vi "Init.vi"(8 "error in":errorcluster) -> (0 "error out":errorcluster)   [LabVIEW 2018, in "UDP Writer.lvlib"]
doc: "This subVI enqueues the named action in to the communications queue along with the input data."
uses:
  UDP Writer.lvlib
  Private Controls/Module Data.ctl
  Private Controls/Module Action.ctl
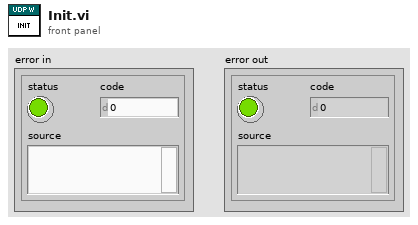
[diagram p1: front panel]
types:
  T1 = typedef "UDP Writer.lvlib/Module Data.ctl" = cluster{"Data":variant, "Action":T2}
  T2 = typedef "UDP Writer.lvlib/Module Action.ctl" = enum16{"Init", "Update ARINC", "Update Waterfall", "Update RPMs", "Update Temps", "Update Modbus", "Update AI", "Update Vibs", "Write", "Error"}
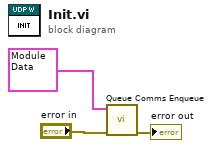
[diagram p0: block diagram]
diagram:
  n1 = call "Queue Comms Enqueue.vi"("error in (no error)"="error in", "element"=T1 {"Data"=variant, "Action"=enum."Init"}) -> ("error out"=→"error out":errorcluster)  [unwired: 9 in]
